vi "XYZ Coordinate to String.vi"(1 "Coordinate Control":T1) -> (0 "String":string)   [LabVIEW 2014]
uses:
  XYZ Coordinate Control.ctl
panel:
  # "LICENSED MATERIALS – PROPERTY OF IBM\nCopyright IBM Corp. 2016,\nALL RIGHTS RESERVED"
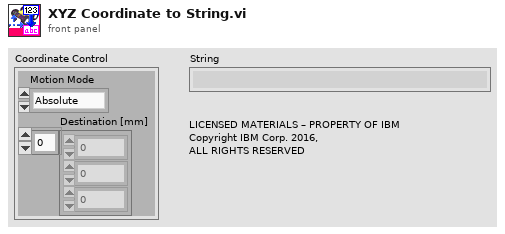
[diagram p1: front panel]
types:
  T1 = typedef "XYZ Coordinate Control.ctl" = cluster{"Motion Mode":enum16{"Absolute", "Relative"}, "Destination [mm]":dbl[]}
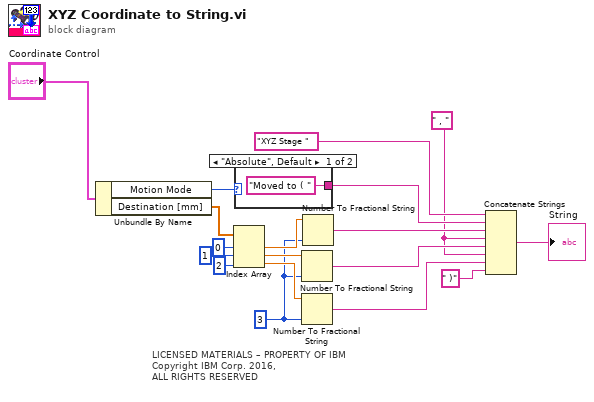
[diagram p0: block diagram]
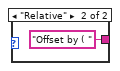
[diagram p2: hidden frame]
diagram:
  w1 = i16 3 ("precision (6)")
  w4 = " , " ("string")
  # "LICENSED MATERIALS – PROPERTY OF IBM\nCopyright IBM Corp. 2016,\nALL RIGHTS RESERVED"
  n1 = Unbundle By Name("Coordinate Control") -> ("Motion Mode"=w7:enum16{"Absolute", "Relative"}, "Destination [mm]"=w11:dbl[])
  n2 = Index Array(array=w11, index #1=0 ("index"), index #2=1 ("index"), index #3=2 ("index")) -> (element #1=w15:dbl, element #2=w16:dbl, element #3=w17:dbl)
  n3 = case shown="\"Absolute\", Default" w7 {
    tunnel: ["Moved to ( " ("button name (\"OK\")") "Offset by ( " ("button name (\"OK\")")] -> w9
    frame "Absolute", Default {
    }
    frame "Relative" {
    }
  }
  n4 = Number To Fractional String(number=w16, precision (6)=w1) -> (F-format string=w5:string)  [unwired: 2 in]
  n5 = Number To Fractional String(number=w17, precision (6)=w1) -> (F-format string=w3:string)  [unwired: 2 in]
  n6 = Number To Fractional String(number=w15, precision (6)=w1) -> (F-format string=w18:string)  [unwired: 2 in]
  n7 = Concatenate Strings("XYZ Stage " ("button name (\"OK\")"), w9, w18, w4, w5, w4, w3, " )" ("string")) -> (→"String":string)
